vi "Add Model_Add.vi"(8 "error in (no error)":errorcluster, 9 "Settings":T1, 11 "Model Ref":refnum<k24>) -> (0 "error out":errorcluster, 3 "Model Ref Out":refnum<k24>)   [LabVIEW 2019, in "Simple SysDef API.lvlib"]
uses:
  <userlib>/SimpleSysDef/Simple SysDef API.lvlib
  NationalInstruments.VeriStand.SystemDefinitionAPI
  <userlib>/SimpleSysDef/_SubVIs/Add Model_Settings.ctl
  NationalInstruments.VeriStand.SystemStorage
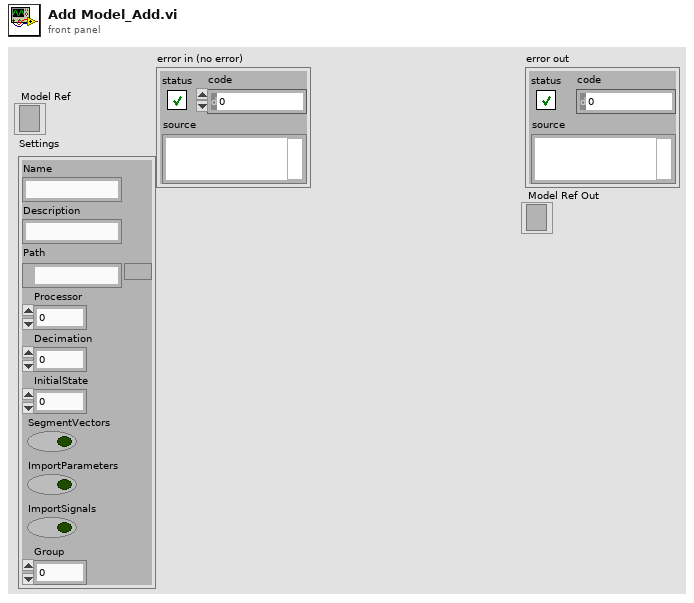
[diagram p1: front panel]
types:
  T1 = typedef "Simple SysDef API.lvlib/Add Model_Settings.ctl" = cluster{"Name":string, "Description":string, "Path":path, "Processor":i32, "Decimation":i32, "InitialState":u16, "SegmentVectors":bool, "ImportParameters":bool, "ImportSignals":bool, "Group":i32}
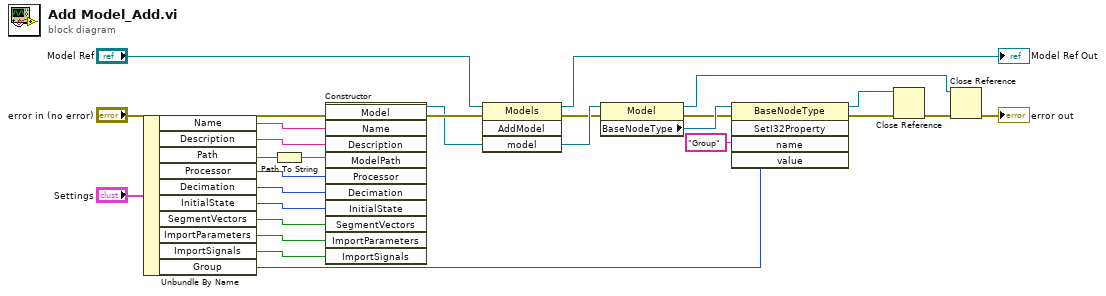
[diagram p0: block diagram]
diagram:
  n1 = Unbundle By Name("Settings") -> ("Name"=w22:string, "Description"=w21:string, "Path"=w20:path, "Processor"=w19:i32, "Decimation"=w18:i32, "InitialState"=w17:u16, "SegmentVectors"=w16:bool, "ImportParameters"=w15:bool, "ImportSignals"=w14:bool, "Group"=w1:i32)
  n2 = Path To String(path=w20) -> (string=w24:string)
  n3 = constructor class="Model"(error in="error in (no error)", "Name"=w22, "Description"=w21, "ModelPath"=w24, "Processor"=w19, "Decimation"=w18, "InitialState"=w17, "SegmentVectors"=w16, "ImportParameters"=w15, "ImportSignals"=w14) -> (reference out=w7:refnum<k24>, error out=w25:errorcluster)  [unwired: 2 in, 10 out]
  n4 = invoke class="Models" method="AddModel"(reference="Model Ref", error in=w25, "model"=w7) -> (reference out=→"Model Ref Out":refnum<k24>, error out=w5:errorcluster)  [unwired: 1 in, 2 out]
  n5 = property class="Model"(reference=w7, error in=w5) -> (reference out=w6:refnum<k24>, error out=w9:errorcluster, "BaseNodeType"=w10:refnum<k24>)
  n6 = invoke class="BaseNodeType" method="SetI32Property"(reference=w10, error in=w9, "name"="Group", "value"=w1) -> (reference out=w2:refnum<k24>, error out=w4:errorcluster)  [unwired: 1 in, 3 out]
  n7 = Close Reference(reference=w2, error in (no error)=w4) -> (error out=w3:errorcluster)
  n8 = Close Reference(reference=w6, error in (no error)=w3) -> (error out=→"error out":errorcluster)
